vi "Launch PPMS UI.vi"() -> ()   [LabVIEW 2016, in "Instrument.PPMS UI.lvclass"]
doc: "This will launch a stan-alone user interface for the PPMS 2 Instrument\n\nJKI State Machine Objects (SMO) 1.0.0.5\nJKI - JKI\nCopyright (c) 2016, JKI"
uses:
  Instrument.PPMS UI.lvclass
  C:/Program Files (x86)/National Instruments/LabVIEW 2016/vi.lib/JKI/JKI SMO/SMO/SMO.lvclass
  C:/Program Files (x86)/National Instruments/LabVIEW 2016/vi.lib/JKI/JKI SMO/SMO.UI/SMO.UI.lvclass
  instrument.PPMS/instrument.PPMS.lvclass
  C:/Program Files (x86)/National Instruments/LabVIEW 2016/user.lib/LevyLab/Levylab Instruments/SMOs/Instrument/Instrument.lvclass
  <userlib>/LevyLab/Levylab Instruments/SMOs/Instrument/Typedefs/SMO Configuration--Cluster.ctl
  <userlib>/LevyLab/Levylab Instruments/SMOs/Instrument/Typedefs/SMO RC Type--enum.ctl
  <userlib>/LevyLab/Levylab Instruments/SMOs/Instrument/Instrument.lvclass/Instrument.ctl
  Instrument.PPMS UI.lvclass/Instrument.PPMS UI.ctl
  <vilib>/JKI/JKI SMO/SMO/Typedefs/SMOState --Enum.ctl
  <vilib>/JKI/JKI SMO/SMO/SMO.lvclass
  <vilib>/JKI/JKI SMO/SMO.UI/SMO.UI.lvclass
  <userlib>/LevyLab/Levylab Instruments/SMOs/Instrument/Instrument.lvclass
panel:
  in  "Address":string
  out "error out":errorcluster
  in  "Stop":bool
  # "Launch PPMS 2 UI"
  # "For instructions on how to use the JKI State Machine Objects, examples and video tutorials, visit:\nhttp://jki.net/state-machine-objects/\n\nJKI State Machine Objects™\nhttp://jki.net/state-machine-objects/\nCopyright (C) 2005-2015, JKI <info@jki.net>\nALL RIGHTS RESERVED"
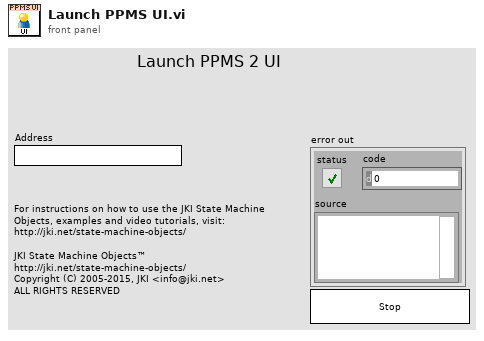
[diagram p1: front panel]
types:
  T1 = typedef "Instrument.lvclass/SMO RC Type--enum.ctl" = enum16{"RC", "STM", "ZMQ"}
  T2 = typedef "Instrument.lvclass/SMO Configuration--Cluster.ctl" = cluster{"Address":string, "Port":u16, "RC Type":T1}
  T3 = typedef "SMO.lvclass/Public Events.ctl" = cluster{"Error":refnum<user-event>, "State":refnum<user-event>, "Reserve State":refnum<user-event>}
  T4 = typedef "SMO.UI.lvclass/PublicEvents--Cluster.ctl" = cluster{"UI Hidden":refnum<user-event>, "UI State":refnum<user-event>}
  T5 = typedef "SMO.lvclass/SMOState --Enum.ctl" = enum16{"unknown", "Created", "Started", "Stopped"}
  T6 = enum32{"Invalid", "Standard", "Closed", "Hidden", "Minimized", "Maximized"}
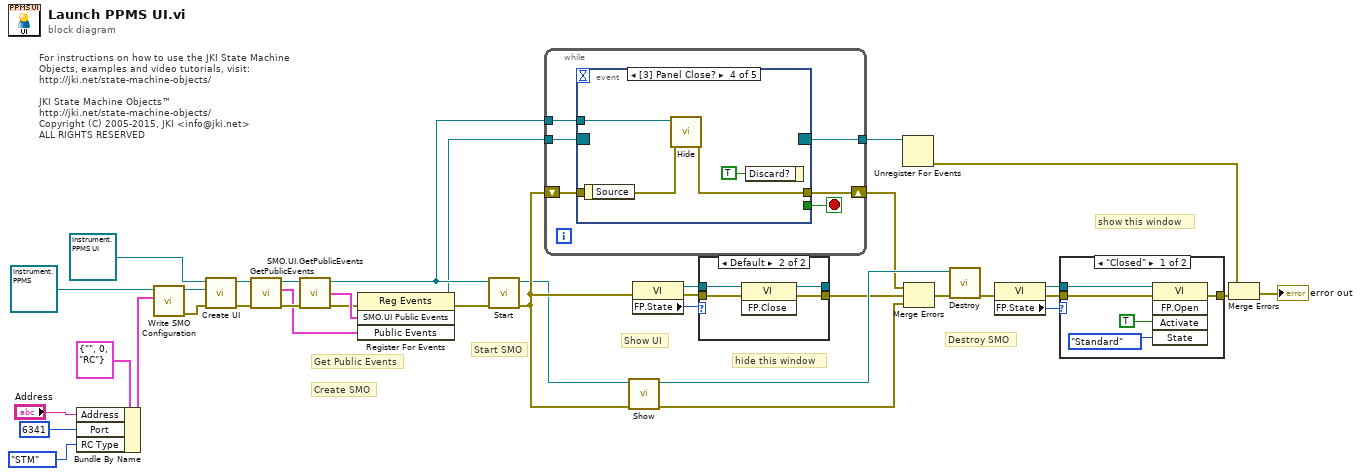
[diagram p0: block diagram]
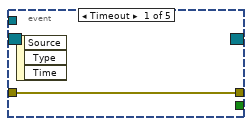
[diagram p4: hidden frame]
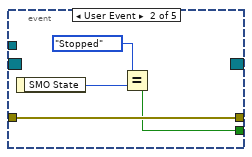
[diagram p5: hidden frame]
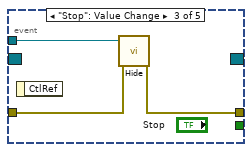
[diagram p6: hidden frame]
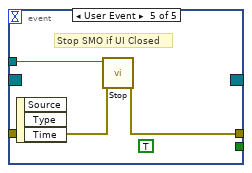
[diagram p7: hidden frame]
diagram:
  # "show this window"
  # "hide this window"
  # "Show UI"
  # "For instructions on how to use the JKI State Machine Objects, examples and video tutorials, visit:\nhttp://jki.net/state-machine-objects/\n\nJKI State Machine Objects™\nhttp://jki.net/state-machine-objects/\nCopyright (C) 2005-2015, JKI <info@jki.net>\nALL RIGHTS RESERVED"
  # "Get Public Events"
  # "Start SMO"
  # "Destroy SMO"
  # "Create SMO"
  n1 = Bundle By Name(cluster=T2 {"Address"="", "Port"=0, "RC Type"=enum."RC"} ("SMO"), "Address"="Address", "Port"=6341, "RC Type"=SMO_RC_Type--enum."STM") -> (w5:T2)
  n2 = call <userlib>:"Write SMO Configuration.vi"("SMO"=w5, "Instrument in"=refnum<class "instrument.PPMS.lvclass"> refnum ("instrument.PPMS.lvclass")) -> ("error out"=w1:errorcluster, "Instrument out"=w22:refnum<class "instrument.PPMS.lvclass">)  [unwired: 8 in]
  n3 = call "Create UI.vi"("error in (no error)"=w1, "instrument.PPMS.lvclass"=w22, "Instrument.PPMS UI in"=refnum<class "Instrument.PPMS UI.lvclass"> refnum ("SMO.Template.lvclass")) -> ("error out"=w24:errorcluster, "Instrument.PPMS UI out"=w23:refnum<class "Instrument.PPMS UI.lvclass">)  [unwired: 7 in]
  n4 = call <vilib>:"GetPublicEvents.vi"("error in (no error)"=w24, "SMO"=w23) -> ("error out"=w26:errorcluster, "Public Events"=w25:T3, "SMO out"=w27:refnum<class "Instrument.PPMS UI.lvclass">)  [unwired: 7 in]
  n5 = call <vilib>:"SMO.UI.GetPublicEvents.vi"("error in (no error)"=w26, "SMO.UI"=w27) -> ("error out"=w30:errorcluster, "SMO.UI Public Events"=w31:T4, "SMO.UI out"=w32:refnum<class "Instrument.PPMS UI.lvclass">)  [unwired: 7 in]
  n6 = register-events(error in=w30, w31, w25) -> (reference out=w28:refnum<event-registration>, error out=w29:errorcluster)  [unwired: 1 in]
  n7 = call <vilib>:"Start.vi"("error in (no error)"=w29, "SMO"=w32) -> ("error out"=w18:errorcluster, "SMO out"=w6:refnum<class "Instrument.PPMS UI.lvclass">)  [unwired: 8 in]
  n8 = while {
    shift-right: [w42] -> w8
    shift-left: w18 -> [w41]
    tunnel: w28 -> [w40]
    tunnel: [w39] -> w37
    tunnel: w32 -> [w38]
    stop <- w43 stop-if-true
    n9 = event shown="[3] Panel Close?" {
      selector: w40 -> [_ _ _ _ _]
      dyn-events: [_ _ _ _ _] -> w39
      timeout: _ -> [_ _ _ _ _]
      tunnel: [_ w45 _ _ _] -> w43
      tunnel: w38 -> [_ _ w51 w54 w58]
      tunnel: [w44 w48 w49 w52 w57] -> w42
      tunnel: w41 -> [w44 w48 w50 w53 w56]
      event Timeout {
        n10 = event-data() -> ()  [unwired: 1 in, 3 out]
      }
      event User Event {
        n11 = event-data() -> ("SMO State"=w47:T5)  [unwired: 1 in]
        n12 = Equal?(x=SMOState_--Enum."Stopped", y=w47) -> (x = y?=w45:bool)
      }
      event "Stop": Value Change {
        n13 = event-data() -> ()  [unwired: 1 in, 1 out]
        n14 = call <vilib>:"Hide.vi"("error in (no error)"=w50, "SMO.UI"=w51) -> ("error out"=w49:errorcluster)  [unwired: 8 in, 1 out]
      }
      event Panel Close? {
        n15 = event-data() -> ()  [unwired: 1 in, 1 out]
        n16 = call <vilib>:"Hide.vi"("error in (no error)"=w53, "SMO.UI"=w54) -> ("error out"=w52:errorcluster)  [unwired: 8 in, 1 out]
        n17 = event-data("Discard?"=TRUE ("OK")) -> ()  [unwired: 1 in, 1 out]
      }
      event User Event {
        (unwired) TRUE ("OK")
        # "Stop SMO if UI Closed"
        n18 = event-data() -> ()  [unwired: 1 in, 3 out]
        n19 = call <vilib>:"Stop.vi"("error in (no error)"=w56, "SMO"=w58) -> ("error out"=w57:errorcluster)  [unwired: 8 in, 1 out]
      }
    }
  }
  n20 = call <vilib>:"Show.vi"("error in (no error)"=w18, "SMO.UI"=w6) -> ("error out"=w7:errorcluster, "SMO.UI out"=w34:refnum<class "Instrument.PPMS UI.lvclass">)  [unwired: 8 in]
  n21 = property class="VI"(error in=w18) -> (reference out=w16:refnum<vi>, error out=w17:errorcluster, "FP.State"=w15:T6)  [unwired: 1 in]
  n22 = case shown="Default" w15 {
    tunnel: [w60 w64] -> w9
    tunnel: w17 -> [w60 w63]
    tunnel: w16 -> [w59 w62]
    tunnel: [w59 w61] -> _
    frame "Invalid", "Closed" {
    }
    frame Default {
      n23 = invoke class="VI" method="FP.Close"(reference=w62, error in=w63) -> (reference out=w61:refnum<vi>, error out=w64:errorcluster)  [unwired: 1 in, 1 out]
    }
  }
  n24 = Unregister For Events(event registration refnum=w37) -> (error out=w36:errorcluster)  [unwired: 1 in]
  n25 = Merge Errors(w8, w9, w7) -> (w33:errorcluster)
  n26 = call <vilib>:"Destroy.vi"("error in (no error)"=w33, "SMO"=w34) -> ("error out"=w11:errorcluster)  [unwired: 9 in]
  n27 = property class="VI"(error in=w11) -> (reference out=w12:refnum<vi>, error out=w13:errorcluster, "FP.State"=w14:T6)  [unwired: 1 in]
  n28 = case shown="\"Closed\"" w14 {
    tunnel: [w67 w70] -> w10
    tunnel: w13 -> [w66 w70]
    tunnel: w12 -> [w65 _]
    frame "Closed" {
      n29 = invoke class="VI" method="FP.Open"(reference=w65, error in=w66, "Activate"=TRUE, "State"=T6."Standard") -> (error out=w67:errorcluster)  [unwired: 1 in, 4 out]
    }
    frame Default {
    }
  }
  n30 = Merge Errors(w36, w10) -> (→"error out":errorcluster)
